vi "Command.vi"(7 "additional timeout, ms (0)":u32, 8 "error in (no error)":errorcluster, 9 "data":cluster{"offset":u32, "data":u8[]}[](array[cluster]), 10 "command":u8, 11 "SOL Camera in":refnum<class "PL SOL Instruments Camera.lvclass">) -> (0 "error out":errorcluster, 2 "response":u8[](array[numeric]), 3 "SOL Camera out":refnum<class "PL SOL Instruments Camera.lvclass">)   [LabVIEW 2015, in "PL SOL Instruments Camera.lvclass"]
doc: "Sends <b>command</b> and <b>data</b> to device and returns <b>response</b>."
uses:
  PL SOL Instruments Camera.lvclass
  PL SOL Instruments Camera.lvclass/PL SOL Instruments Camera.ctl
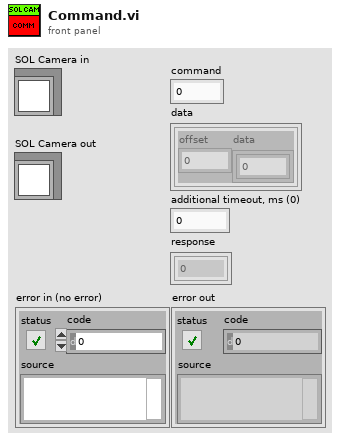
[diagram p1: front panel]
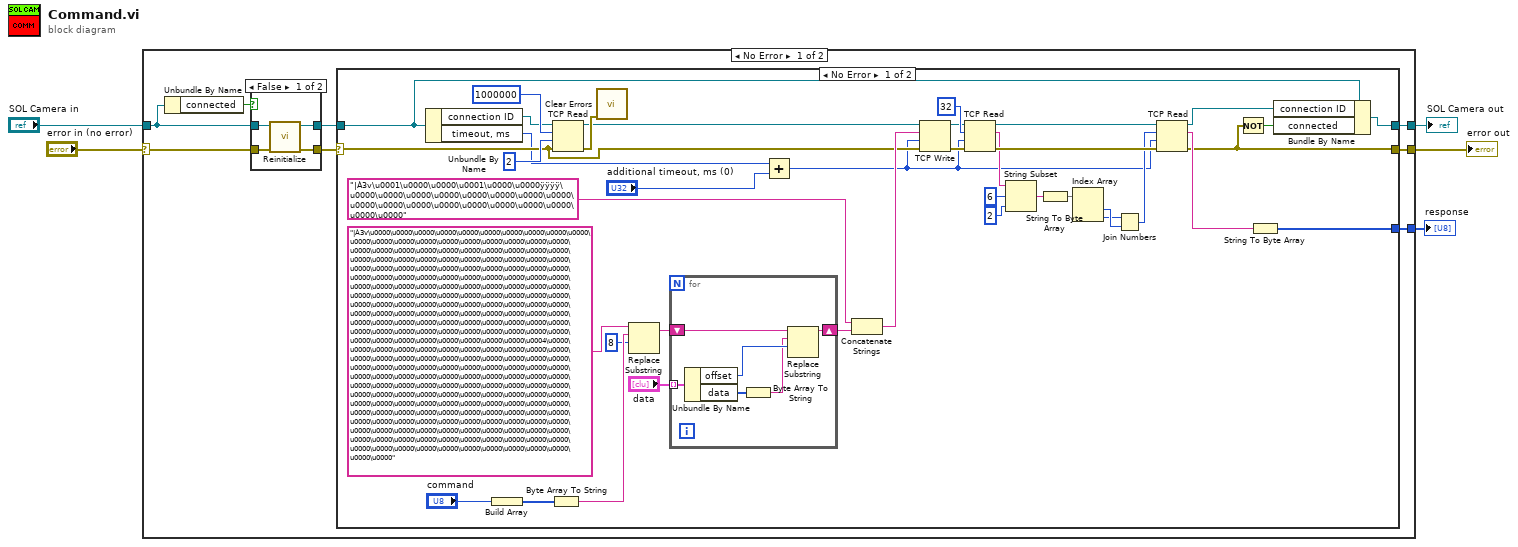
[diagram p0: block diagram]
diagram:
  n1 = case shown="No Error" "error in (no error)" {
    selector: "error in (no error)" -> [w11 w68]
    tunnel: "SOL Camera in" -> [w12 w67]
    tunnel: [w8 w68] -> w2
    tunnel: [w7 w67] -> w3
    tunnel: [w6 _] -> w1
    frame No Error {
      n2 = Unbundle By Name(w12) -> ("connected"=w13:bool)
      n3 = case shown="False" w13 {
        tunnel: w12 -> [w64 w66]
        tunnel: w11 -> [w63 w65]
        tunnel: [w62 w66] -> w9
        tunnel: [w61 w65] -> w10
        frame False {
          n4 = call "Reinitialize.vi"("error in (no error)"=w63, "SOL MS in"=w64) -> ("error out"=w61:errorcluster, "SOL Camera out"=w62:refnum<class "PL SOL Instruments Camera.lvclass">)  [unwired: 8 in]
        }
        frame True {
        }
      }
      n5 = case shown="No Error" w10 {
        selector: w10 -> [w22 w60]
        tunnel: w9 -> [w23 w59]
        tunnel: [w17 w60] -> w8
        tunnel: [w16 w59] -> w7
        tunnel: [w15 _] -> w6
        frame No Error {
          n6 = Unbundle By Name(w23) -> ("connection ID"=w48:refnum<k5>, "timeout, ms"=w20:u32)
          n7 = Build Array("command") -> (w25:u8[])
          n8 = Byte Array To String(unsigned byte array=w25) -> (string=w26:string)
          n9 = TCP Read(connection ID=w48, bytes to read=1000000, error in (no error)=w22, 9:2 ("timeout ms (25000)")) -> (connection ID out=w49:refnum<k5>, error out=w50:errorcluster)  [unwired: 1 in, 1 out]
          n10 = call <vilib>:"Clear Errors.vi"("error in (no error)"=w50) -> ()  [unwired: 5 in, 2 out]
          n11 = Replace Substring(3:8 ("offset (0)"), 4:w26, 5:"|À3v\u0000\u0000\u0000\u0000\u0000\u0000\u0000\u0000\u0000\u0000\u0000\u0000\u0000\u0000\u0000\u0000\u0000\u0000\u0000\u0000\u0000\u0000\u0000\u0000\u0000\u0000\u0000\u0000\u0000\u0000\u0000\u0000\u0000\u0000\u0000\u0000\u0000\u0000\u0000\u0000\u0000\u0000\u0000\u0000\u0000\u0000\u0000\u0000\u0000\u0000\u0000\u0000\u0000\u0000\u0000\u0000\u0000\u0000\u0000\u0000\u0000\u0000\u0000\u0000\u0000\u0000\u0000\u0000\u0000\u0000\u0000\u0000\u0000\u0000\u0000\u0000\u0000\u0000\u0000\u0000\u0000\u0000\u0000\u0000\u0000\u0000\u0000\u0000\u0000\u0000\u0000\u0000\u0000\u0000\u0000\u0000\u0000\u0000\u0000\u0000\u0000\u0000\u0000\u0000\u0000\u0000\u0000\u0000\u0000\u0000\u0000\u0000\u0000\u0000\u0000\u0000\u0000\u0000\u0000\u0000\u0000\u0000\u0000\u0000\u0000\u0000\u0000\u0000\u0004\u0000\u0000\u0000\u0000\u0000\u0000\u0000\u0000\u0000\u0000\u0000\u0000\u0000\u0000\u0000\u0000\u0000\u0000\u0000\u0000\u0000\u0000\u0000\u0000\u0000\u0000\u0000\u0000\u0000\u0000\u0000\u0000\u0000\u0000\u0000\u0000\u0000\u0000\u0000\u0000\u0000\u0000\u0000\u0000\u0000\u0000\u0000\u0000\u0000\u0000\u0000\u0000\u0000\u0000\u0000\u0000\u0000\u0000\u0000\u0000\u0000\u0000\u0000\u0000\u0000\u0000\u0000\u0000\u0000\u0000\u0000\u0000\u0000\u0000\u0000\u0000\u0000\u0000\u0000\u0000\u0000\u0000\u0000\u0000\u0000\u0000\u0000\u0000\u0000\u0000\u0000\u0000\u0000\u0000\u0000\u0000\u0000\u0000\u0000\u0000\u0000\u0000\u0000\u0000\u0000\u0000\u0000\u0000\u0000\u0000\u0000\u0000\u0000\u0000\u0000\u0000\u0000\u0000\u0000\u0000\u0000\u0000\u0000") -> (1:w27:string)  [unwired: 1 in, 1 out]
          n12 = for {
            shift-right: [w54] -> w28
            shift-left: w27 -> [w57]
            tunnel: "data" -> [w58] mode=indexing
            n13 = Unbundle By Name(w58) -> ("offset"=w56:u32, "data"=w55:u8[])
            n14 = Byte Array To String(unsigned byte array=w55) -> (string=w53:string)
            n15 = Replace Substring(3:w56, 4:w53, 5:w57) -> (1:w54:string)  [unwired: 1 in, 1 out]
          }
          n16 = Add(x=w20, y="additional timeout, ms (0)") -> (x+y=w18:u32)
          n17 = Concatenate Strings("|À3v\u0001\u0000\u0000\u0001\u0000\u0000ÿÿÿÿ\u0000\u0000\u0000\u0000\u0000\u0000\u0000\u0000\u0000\u0000\u0000\u0000\u0000\u0000\u0000\u0000\u0000\u0000", w28) -> (w46:string)
          n18 = TCP Write(connection ID=w49, data in=w46, error in (no error)=w22, 9:w18) -> (connection ID out=w29:refnum<k5>, error out=w30:errorcluster)  [unwired: 1 out]
          n19 = TCP Read(connection ID=w29, bytes to read=32, error in (no error)=w30, 9:w18) -> (connection ID out=w40:refnum<k5>, data out=w32:string, error out=w42:errorcluster)  [unwired: 1 in]
          n20 = String Subset(string=w32, offset (0)=6, length (rest)=2 ("length (rest)")) -> (substring=w35:string)
          n21 = String To Byte Array(string=w35) -> (unsigned byte array=w36:u8[])
          n22 = Index Array(array=w36) -> (element #1=w38:u8, element #2=w37:u8)  [unwired: 2 in]
          n23 = Join Numbers(hi=w37, lo=w38) -> ((hi.lo)=w39:u16)
          n24 = TCP Read(connection ID=w40, bytes to read=w39, error in (no error)=w42, 9:w18) -> (connection ID out=w41:refnum<k5>, data out=w44:string, error out=w17:errorcluster)  [unwired: 1 in]
          n25 = Not(x=w17) -> (.not. x?=w43:bool)
          n26 = String To Byte Array(string=w44) -> (unsigned byte array=w15:u8[])
          n27 = Bundle By Name(cluster=w23, "connection ID"=w41, "connected"=w43) -> (w16:refnum<class "PL SOL Instruments Camera.lvclass">)
        }
        frame Error {
        }
      }
    }
    frame Error {
    }
  }
  "SOL Camera out" <- w3
  "error out" <- w2
  "response" <- w1
